vi "Cursor.Manage.vi"(6 "VI reference (current VI)":refnum<vi>, 8 "error in (no error)":errorcluster, 11 "Cmd list":string[](array[string])) -> (0 "error out":errorcluster)   [LabVIEW 2015, in "Simple Sequence Tools - Editor.lvlib"]
uses:
  Simple Sequence Tools - Editor.lvlib
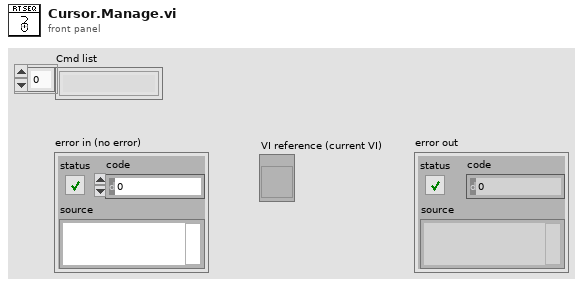
[diagram p1: front panel]
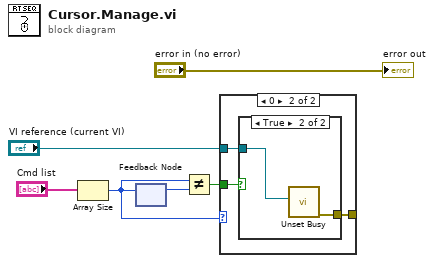
[diagram p0: block diagram]
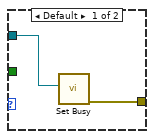
[diagram p2: hidden frame]
diagram:
  n1 = Array Size(array="Cmd list") -> (size(s)=w4:i32)
  n2 = feedback #1(w4) -> (w5:i32)
  n3 = feedback-in #1(w4) -> ()
  n4 = Not Equal?(x=w4, y=w5) -> (x != y?=w3:bool)
  n5 = case shown="0" w4 {
    tunnel: w3 -> [_ w11]
    tunnel: [w8 w10] -> _
    tunnel: "VI reference (current VI)" -> [w7 w9]
    frame Default {
      n6 = call <vilib>:"Set Busy.vi"("VI reference (current VI)"=w7) -> ("error out"=w8:errorcluster)  [unwired: 9 in, 1 out]
    }
    frame 0 {
      n7 = case shown="True" w11 {
        tunnel: [_ w13] -> w10
        tunnel: w9 -> [_ w12]
        frame False {
        }
        frame True {
          n8 = call <vilib>:"Unset Busy.vi"("VI reference (current VI)"=w12) -> ("error out"=w13:errorcluster)  [unwired: 10 in]
        }
      }
    }
  }
  "error out" <- "error in (no error)"
